vi "measure voltage_2 sub test.vi"(8 "error in (no error)":errorcluster, 11 "VISA Refnum in":refnum<visa-resource-name>) -> (0 "error out":errorcluster, 3 "Reponse":string)   [LabVIEW 2024]
uses:
  C:/Program Files/National Instruments/LabVIEW 2024/examples/Instrument IO/Serial/support/Serial - Settings.ctl
  C:/Program Files/National Instruments/LabVIEW 2024/examples/Instrument IO/Serial/support/Serial - XON-XOFF Characters.ctl
  C:/Program Files/National Instruments/LabVIEW 2024/examples/Instrument IO/Serial/support/Serial - ASCII Characters.ctl
  <vilib>/Instr/_visa.llb/VISA Configure Serial Port (Instr).vi
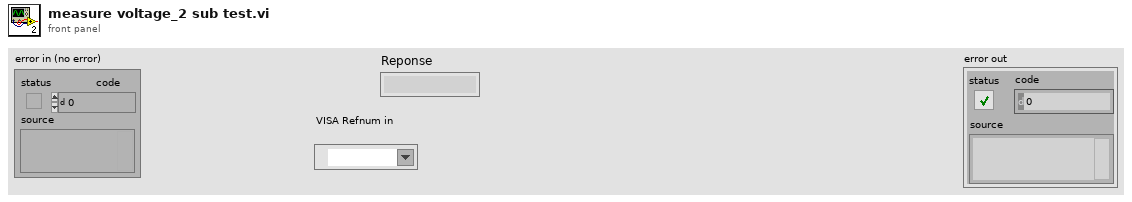
[diagram p1: front panel]
types:
  T1 = typedef "Serial - XON-XOFF Characters.ctl" = cluster{"XON":T2, "XOFF":T2}
  T2 = typedef "Serial - ASCII Characters.ctl" = enum16{"NUL", "SOH", "STX", "ETX", "EOT", "ENQ", "ACK", "BEL", "BS", "HT", "LF", "VT", "FF", "CR", "SO", "SI", "DLE", "DC1", "DC2", "DC3", "DC4", "NAK", "SYN", "ETB", "CAN", "EM", "SUB", "ESC", "FS", "GS", "RS", "US", "SP", "!", "\"", "#", "$", "%", "&", "'", "(", ")", "*", "+", ",", "- (-)", ".", "/", "0", "1", "2", "3", "4", "5", "6", "7", "8", "9", ":", ";", "<", "=", ">", "?", "@", "A", "B", "C", "D", "E", "F", "G", "H", "I", "J", "K", "L", "M", "N", "O", "P", "Q", "R", "S", "T", "U", "V", "W", "X", "Y", "Z", "[", "\\", "]", "^", "_", "`", "a", "b", "c", "d", "e", "f", "g", "h", "i", "j", "k", "l", "m", "n", "o", "p", "q", "r", "s", "t", "u", "v", "w", "x", "y", "z", "{", "|", "}", "~"}
  T3 = typedef "Serial - Settings.ctl" = cluster{"baud rate":u32, "data bits":u16, "parity":enum16{"None", "Odd", "Even", "Mark", "Space"}, "stop bits":u16, "flow control":u16}
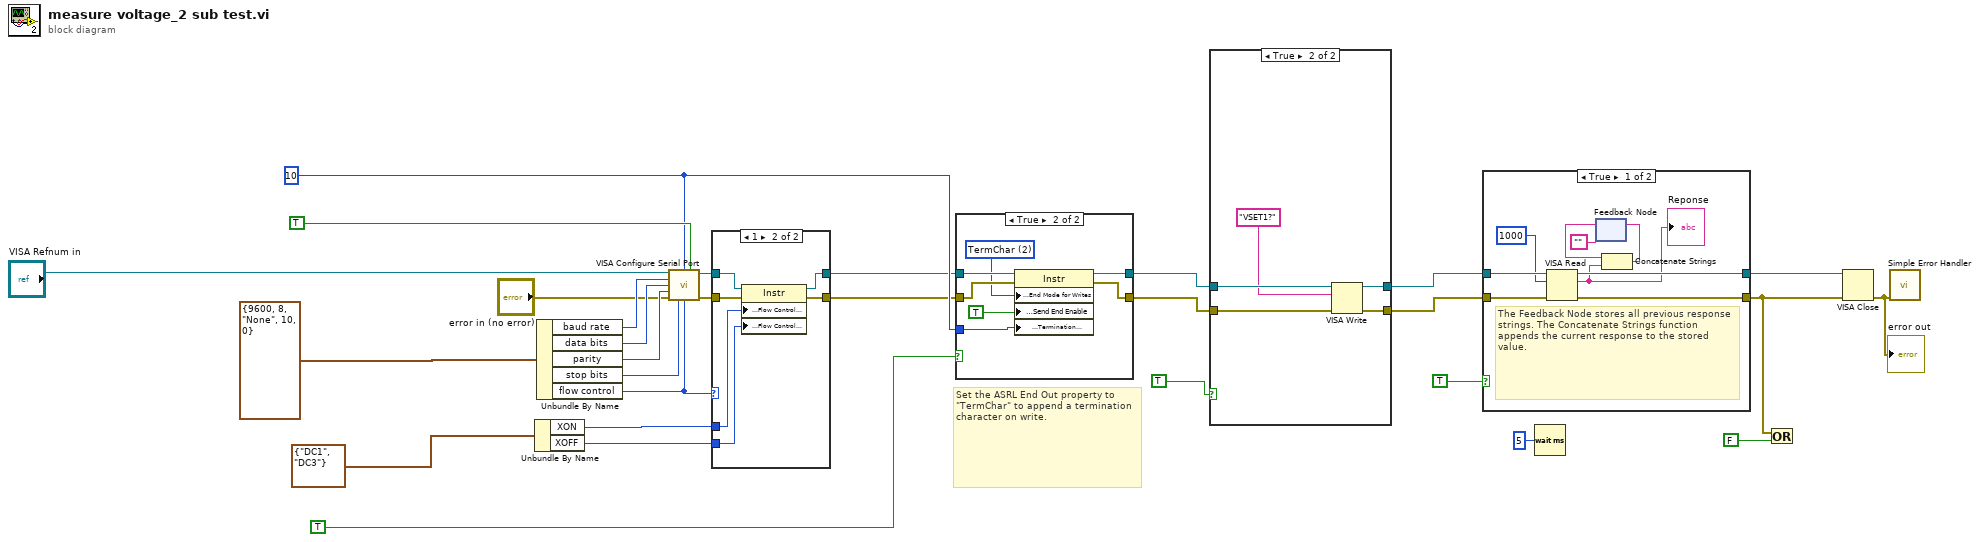
[diagram p0: block diagram]
diagram:
  w24 = u8 10 ("Termination Character")
  # "Set the ASRL End Out property to \"TermChar\" to append a termination character on write."
  n1 = Unbundle By Name(T1 {"XON"=enum."DC1", "XOFF"=enum."DC3"} ("XON/XOFF Characters 2")) -> ("XON"=w12:T2, "XOFF"=w11:T2)
  n2 = Unbundle By Name(T3 {"baud rate"=9600, "data bits"=8, "parity"=enum."None", "stop bits"=10, "flow control"=0} ("Serial Settings 2")) -> ("baud rate"=w17:u32, "data bits"=w18:u16, "parity"=w19:enum16{"None", "Odd", "Even", "Mark", "Space"}, "stop bits"=w20:u16, "flow control"=w13:u16)
  n3 = call-poly "VISA Configure Serial Port"("VISA resource name"="VISA Refnum in", "termination char\n(0xA = '\\n' = LF)"=w24, "Enable Termination\nChar (T)"=TRUE ("End Read on Termination Character?"), "baud rate (9600)"=w17, "data bits (8)"=w18, "parity (0:none)"=w19, "error in (no error)"="error in (no error)", "stop bits (10: 1 bit)"=w20, "flow control (0:none)"=w13) -> ("VISA resource name out"=w21:refnum<visa-resource-name>, "error out"=w22:errorcluster)  [unwired: 1 in, 4 out]
  n4 = case shown="1" w13 {
    tunnel: [w30 w37] -> w10
    tunnel: [w31 w36] -> w8
    tunnel: w22 -> [w30 w35]
    tunnel: w21 -> [w31 w34]
    tunnel: w12 -> [_ w33]
    tunnel: w11 -> [_ w32]
    frame Default {
    }
    frame 1 {
      n5 = property class="Instr"(reference=w34, error in=w35, "Serial Settings:Flow Control XON Character"=w33, "Serial Settings:Flow Control XOFF Character"=w32) -> (reference out=w36:refnum<visa-resource-name>, error out=w37:errorcluster)
    }
  }
  n6 = case shown="True" TRUE ("End Write on Termination Character?") {
    tunnel: w8 -> [w38 w46]
    tunnel: w10 -> [w39 w45]
    tunnel: [w38 w44] -> w7
    tunnel: [w39 w43] -> w9
    tunnel: w24 -> [_ w41]
    frame False {
    }
    frame True {
      w42 = u16 2 items=["None", "LastBit", "TermChar", "Break"] ("Serial Settings:Serial End Mode for Writes")
      n7 = property class="Instr"(reference=w46, error in=w45, "Serial Settings:End Mode for Writes"=w42, "Message Based Settings:Send End Enable"=TRUE, "Message Based Settings:Termination Character"=w41) -> (reference out=w44:refnum<visa-resource-name>, error out=w43:errorcluster)
    }
  }
  n8 = case shown="True" TRUE ("Write 2") {
    tunnel: w7 -> [w48 w53]
    tunnel: w9 -> [w47 w52]
    tunnel: [w48 w51] -> w6
    tunnel: [w47 w50] -> w5
    frame False {
    }
    frame True {
      n9 = VISA Write(VISA resource name=w53, write buffer="VSET1?" ("Command"), error in (no error)=w52) -> (VISA resource name out=w51:refnum<visa-resource-name>, error out=w50:errorcluster)  [unwired: 1 out]
    }
  }
  n10 = case shown="True" TRUE ("Read in") {
    tunnel: [w60 w64] -> w14
    tunnel: w6 -> [w62 w64]
    tunnel: [w58 w63] -> w15
    tunnel: w5 -> [w61 w63]
    frame True {
      # "The Feedback Node stores all previous response strings. The Concatenate Strings function appends the current response to the stored value."
      n11 = VISA Read(VISA resource name=w62, byte count=u32 1000 ("Read Count"), error in (no error)=w61) -> (VISA resource name out=w60:refnum<visa-resource-name>, read buffer=w54:string, error out=w58:errorcluster)  [unwired: 1 out]
      "Reponse" <- w54
      n12 = feedback #1("") -> (w57:string)
      n13 = Concatenate Strings(w57, w54) -> (w55:string)
      n14 = feedback-in #1(w55) -> ()
    }
    frame False {
    }
  }
  n15 = Wait (ms)(milliseconds to wait=u32 5) -> ()  [unwired: 1 out]
  n16 = Or(x=w15, y=FALSE ("Stop")) -> ()  [unwired: 1 out]
  n17 = VISA Close(VISA resource name=w14, error in (no error)=w15) -> (error out=w2:errorcluster)
  "error out" <- w2
  n18 = call <vilib>:"Simple Error Handler.vi"("error in (no error)"=w2) -> ()  [unwired: 1 in, 8 out]
